vi "Finish.vi"   [LabVIEW 2015]
doc: "This VI is called just before exiting. It is expected to close I/O refnum, save collected data, etc."
uses:
  <vilib>/Rock Robotics/WPI/Utilities/WPI_GetSetVariantRefNum.vi
  ADIS16448/ADI MXP IMU/FRC ADI MXP IMU.lvlib
types:
  T1 = typedef "FRC ADI MXP IMU.lvlib/WPI_AnalogDevicesIMUInterruptDevRef.ctl" = cluster{"SimpleGyroDevRef":T2, "InterruptRef":T4}
  T2 = typedef "FRC ADI MXP IMU.lvlib/WPI_AnalogDevicesIMUDevRef.ctl" = cluster{"DevStatus":errorcluster, "Handle":i32, "SPI Bus":T3, "Device Found":bool, "Sample Rate":dbl, "Device Ready":bool, "Yaw Axis":enum16{"X", "Y", "Z"}, "AHRS Algorithm":enum16{"Complementary", "Madgwick"}}
  T3 = typedef "spi_bus.ctl" = enum16{"SPI On-Board, CS0", "SPI On-Board, CS1", "SPI On-Board, CS2", "SPI On-Board, CS3", "SPI MXP", "Invalid"}
  T4 = typedef "WPI_InterruptRef.ctl" = cluster{"DevStatus":errorcluster, "InterruptIndex":T5}
  T5 = typedef "FPGA_InterruptIndex.ctl" = enum8{"0", "1", "2", "3", "4", "5", "6", "7", "Invalid"}
  T6 = typedef "WPI_JoystickDevRef.ctl" = cluster{"Device":T7}
  T7 = typedef "WPI_JoystickDeviceEnum.ctl" = enum16{"USB 0", "USB 1", "USB 2", "USB 3", "USB 4", "USB 5"}
  T8 = typedef "WPI_MotorControlDeviceRef.ctl" = cluster{"DeviceStatus":errorcluster, "Type":T9, "PWM":cluster{"PWM Channel":T10, "DeadBand":T11}, "CAN":cluster{"Device Number":u8, "Control Mode":T12, "Semaphore":T13, "Max Vout":dbl, "TalonSRX Control Mode":T14}, "Invert":bool}
  T9 = typedef "WPI_MotorControlType.ctl" = enum16{"PWM", "CAN", "CANTalonSRX"}
  T10 = typedef "FPGA_DIOPWMChannel.ctl" = enum8{"PWM 0", "PWM 1", "PWM 2", "PWM 3", "PWM 4", "PWM 5", "PWM 6", "PWM 7", "PWM 8", "PWM 9", "PWM MXP 0", "PWM MXP 1", "PWM MXP 2", "PWM MXP 3", "PWM MXP 4", "PWM MXP 5", "PWM MXP 6", "PWM MXP 7", "PWM MXP 8", "PWM MXP 9", "Invalid"}
  T11 = typedef "WPI_PWMDeadband.ctl" = cluster{"Name":string, "maxPositivePwm":i32, "minPositivePwm":i32, "centerPwm":i32, "maxNegativePwm":i32, "minNegativePwm":i32, "angularRange":u16}
  T12 = typedef "WPI_CANJaguar_ControlMode.ctl" = enum8{"Percent VBus", "Current", "Speed", "Position", "Voltage"}
  T13 = typedef "Semaphore RefNum" = refnum<k1>
  T14 = typedef "WPI_CANTalonSRX_APIControlMode.ctl" = enum8{"Percent VBus", "Speed", "Position", "Slave", "Unchanged / Invalid", "Voltage Compensation", "Current", "Motion Profile"}
  T15 = typedef "WPI_CompressorDevRef.ctl" = cluster{"DevStatus":errorcluster, "Pneumatics Control Module":u8}
  T16 = typedef "WPI_EncoderDevRef.ctl" = cluster{"DevStatus":errorcluster, "EncoderIndex":T17, "CounterIndex":T18, "DistancePerCount":dbl, "Decoding Type":T19}
  T17 = typedef "FPGA_EncoderIdx.ctl" = enum8{"Enc 0", "Enc 1", "Enc 2", "Enc 3", "Enc 4", "Enc 5", "Enc 6", "Enc 7", "Invalid"}
  T18 = typedef "FPGA_CounterCtrSystemIndex.ctl" = enum8{"Ctr 0", "Ctr 1", "Ctr 2", "Ctr 3", "Ctr 4", "Ctr 5", "Ctr 6", "Ctr 7", "Invalid"}
  T19 = typedef "WPI_EncoderType.ctl" = enum16{"1x", "2x", "4x"}
  T20 = typedef "WPI_SwitchDevRef.ctl" = cluster{"DevStatus":errorcluster, "DIO Channel":T21, "CntIndex":T18, "Normally Closed":bool}
  T21 = typedef "FPGA_DIOChannel.ctl" = enum8{"DIO 0", "DIO 1", "DIO 2", "DIO 3", "DIO 4", "DIO 5", "DIO 6", "DIO 7", "DIO 8", "DIO 9", "DIO MXP 0", "DIO MXP 1", "DIO MXP 2", "DIO MXP 3", "DIO MXP 4", "DIO MXP 5", "DIO MXP 6", "DIO MXP 7", "DIO MXP 8", "DIO MXP 9", "DIO MXP 10", "DIO MXP 11", "DIO MXP 12", "DIO MXP 13", "DIO MXP 14", "DIO MXP 15", "Invalid"}
  T22 = typedef "WPI_SolenoidDevRef.ctl" = cluster{"DevStatus":errorcluster, "Pneumatics Control Module":u8, "Forward Solenoid Channel":T23, "Reverse Solenoid Channel":T23}
  T23 = typedef "WPI_SolenoidChannel.ctl" = enum8{"Solenoid 0", "Solenoid 1", "Solenoid 2", "Solenoid 3", "Solenoid 4", "Solenoid 5", "Solenoid 6", "Solenoid 7", "Invalid"}
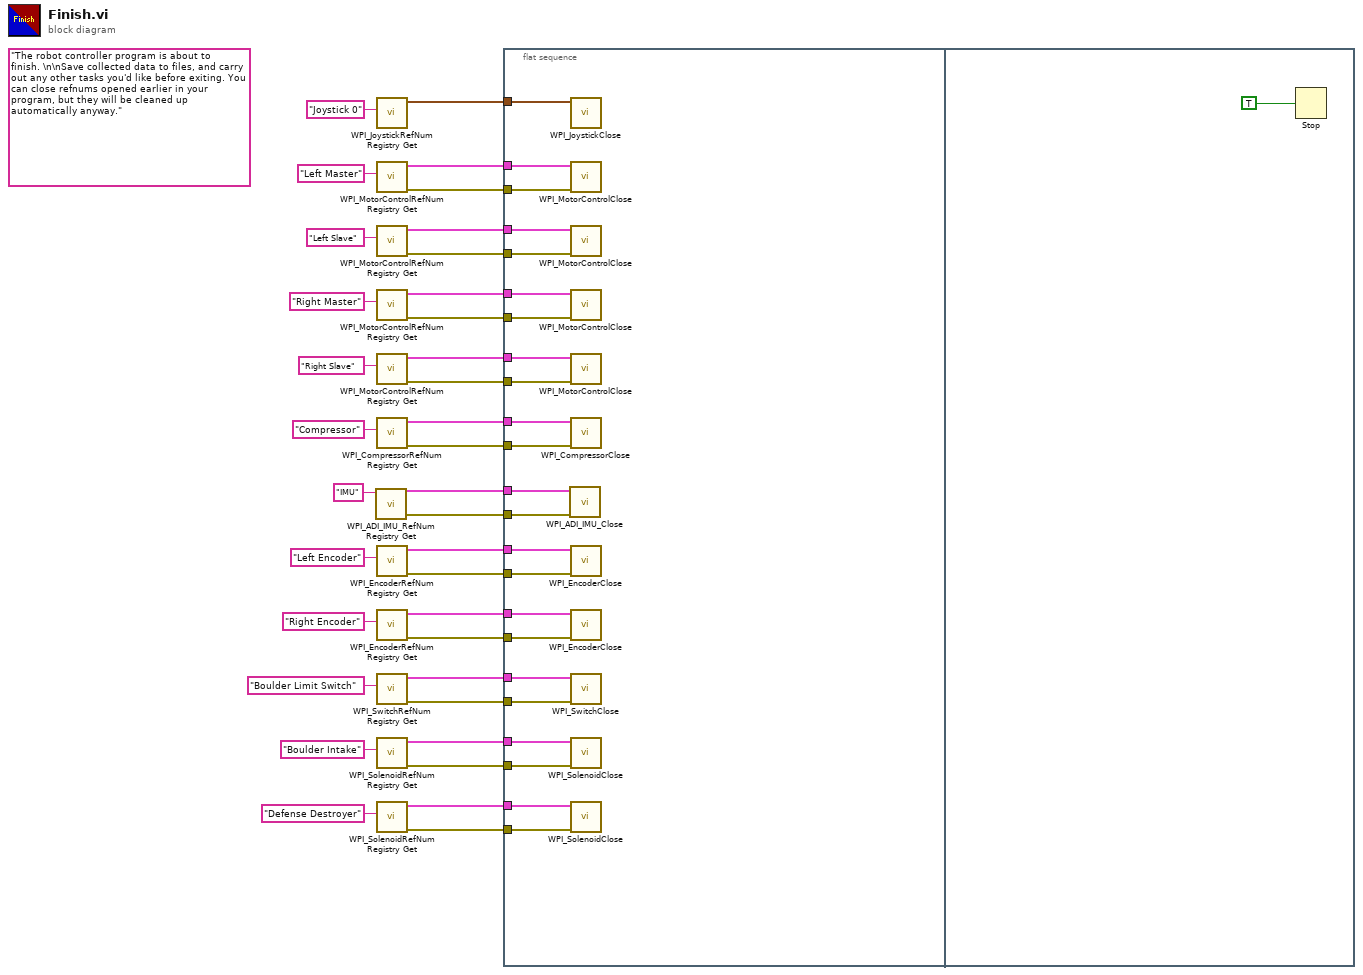
[diagram p0: block diagram]
diagram:
  (unwired) "The robot controller program is about to finish. \n\nSave collected data to files, and carry out any other tasks you'd like before exiting. You can close refnums opened earlier in your program, but they will be cleaned up automatically anyway."
  n1 = call "WPI_ADI_IMU_RefNum Registry Get.vi"("refnum name"="IMU") -> ("error out"=w1:errorcluster, "ADI IMU Interrupt DevRef"=w2:T1)  [unwired: 9 in]
  n2 = call <vilib>:"WPI_JoystickRefNum Registry Get.vi"("refnum name"="Joystick 0") -> ("JoystickDevRef"=w34:T6)  [unwired: 1 in, 9 out]
  n3 = call <vilib>:"WPI_MotorControlRefNum Registry Get.vi"("refnum name"="Left Master") -> ("error out"=w28:errorcluster, "MotorControlDevRef"=w29:T8)  [unwired: 9 in]
  n4 = call <vilib>:"WPI_MotorControlRefNum Registry Get.vi"("refnum name"="Left Slave") -> ("error out"=w26:errorcluster, "MotorControlDevRef"=w27:T8)  [unwired: 9 in]
  n5 = call <vilib>:"WPI_MotorControlRefNum Registry Get.vi"("refnum name"="Right Master") -> ("error out"=w24:errorcluster, "MotorControlDevRef"=w25:T8)  [unwired: 9 in]
  n6 = call <vilib>:"WPI_MotorControlRefNum Registry Get.vi"("refnum name"="Right Slave") -> ("error out"=w22:errorcluster, "MotorControlDevRef"=w23:T8)  [unwired: 9 in]
  n7 = call <vilib>:"WPI_CompressorRefNum Registry Get.vi"("refnum name"="Compressor") -> ("error out"=w20:errorcluster, "CompressorDevRef"=w21:T15)  [unwired: 9 in]
  n8 = call <vilib>:"WPI_EncoderRefNum Registry Get.vi"("refnum name"="Left Encoder") -> ("error out"=w14:errorcluster, "EncoderDevRef"=w15:T16)  [unwired: 9 in]
  n9 = call <vilib>:"WPI_EncoderRefNum Registry Get.vi"("refnum name"="Right Encoder") -> ("error out"=w16:errorcluster, "EncoderDevRef"=w17:T16)  [unwired: 9 in]
  n10 = call <vilib>:"WPI_SwitchRefNum Registry Get.vi"("refnum name"="Boulder Limit Switch") -> ("error out"=w12:errorcluster, "SwitchDevRef"=w13:T20)  [unwired: 9 in]
  n11 = call <vilib>:"WPI_SolenoidRefNum Registry Get.vi"("refnum name"="Boulder Intake") -> ("error out"=w8:errorcluster, "SolenoidDevRef"=w9:T22)  [unwired: 9 in]
  n12 = call <vilib>:"WPI_SolenoidRefNum Registry Get.vi"("refnum name"="Defense Destroyer") -> ("error out"=w5:errorcluster, "SolenoidDevRef"=w6:T22)  [unwired: 9 in]
  n13 = flat-sequence {
    tunnel: w34 -> [w58]
    tunnel: w29 -> [w56]
    tunnel: w28 -> [w57]
    tunnel: w27 -> [w55]
    tunnel: w26 -> [w54]
    tunnel: w25 -> [w53]
    tunnel: w24 -> [w52]
    tunnel: w23 -> [w51]
    tunnel: w22 -> [w50]
    tunnel: w21 -> [w49]
    tunnel: w20 -> [w48]
    tunnel: w17 -> [w47]
    tunnel: w16 -> [w46]
    tunnel: w15 -> [w45]
    tunnel: w14 -> [w44]
    tunnel: w13 -> [w43]
    tunnel: w12 -> [w42]
    tunnel: w9 -> [w41]
    tunnel: w8 -> [w40]
    tunnel: w6 -> [w39]
    tunnel: w5 -> [w38]
    tunnel: w2 -> [w37]
    tunnel: w1 -> [w36]
    frame #0 {
      n14 = call "WPI_ADI_IMU_Close.vi"("error in"=w36, "ADI IMU Interrupt DevRef"=w37) -> ()  [unwired: 9 in, 1 out]
      n15 = call <vilib>:"WPI_JoystickClose.vi"("JoystickDevRef"=w58) -> ()  [unwired: 11 out]
      n16 = call <vilib>:"WPI_MotorControlClose.vi"("error in (no error)"=w57, "MotorControlDevRef"=w56) -> ()  [unwired: 9 in, 1 out]
      n17 = call <vilib>:"WPI_MotorControlClose.vi"("error in (no error)"=w54, "MotorControlDevRef"=w55) -> ()  [unwired: 9 in, 1 out]
      n18 = call <vilib>:"WPI_MotorControlClose.vi"("error in (no error)"=w52, "MotorControlDevRef"=w53) -> ()  [unwired: 9 in, 1 out]
      n19 = call <vilib>:"WPI_MotorControlClose.vi"("error in (no error)"=w50, "MotorControlDevRef"=w51) -> ()  [unwired: 9 in, 1 out]
      n20 = call <vilib>:"WPI_CompressorClose.vi"("error in (no error)"=w48, "CompressorDevRef"=w49) -> ()  [unwired: 9 in, 1 out]
      n21 = call <vilib>:"WPI_EncoderClose.vi"("error in (no error)"=w44, "EncoderDevRef"=w45) -> ()  [unwired: 9 in, 1 out]
      n22 = call <vilib>:"WPI_EncoderClose.vi"("error in (no error)"=w46, "EncoderDevRef"=w47) -> ()  [unwired: 9 in, 1 out]
      n23 = call <vilib>:"WPI_SwitchClose.vi"("error in (no error)"=w42, "SwitchDevRef"=w43) -> ()  [unwired: 9 in, 1 out]
      n24 = call <vilib>:"WPI_SolenoidClose.vi"("error in (no error)"=w40, "SolenoidDevRef"=w41) -> ()  [unwired: 9 in, 1 out]
      n25 = call <vilib>:"WPI_SolenoidClose.vi"("error in (no error)"=w38, "SolenoidDevRef"=w39) -> ()  [unwired: 9 in, 1 out]
    }
    frame #1 {
      n26 = Stop(stop? (T)=TRUE ("Quit")) -> ()
    }
  }
